vi "SetExposure.vi"(8 "error in (no error)":errorcluster, 11 "HamaCam in":refnum<class "HamaCam.lvclass">) -> (0 "error out":errorcluster, 3 "HamaCam out":refnum<class "HamaCam.lvclass">)   [LabVIEW 2023, in "HamaCam.lvlib" / "HamaCam.lvclass"]
uses:
  HamaCam.lvclass
  HamaCam.lvclass/HamaCam.ctl
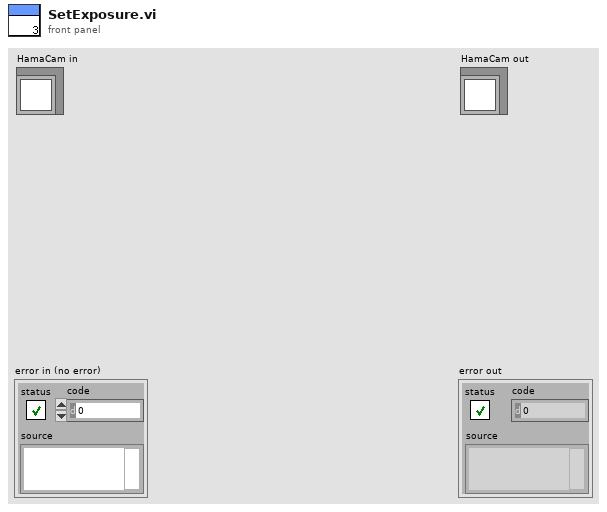
[diagram p1: front panel]
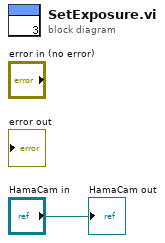
[diagram p0: block diagram]
diagram:
  "HamaCam out" <- "HamaCam in"
